vi "Is Index Visited.vi"(8 "error in (no error)":errorcluster, 10 "Index":i32, 11 "Search in":refnum<class "Search.lvclass">) -> (0 "error out":errorcluster, 2 "Visited?":bool, 3 "Search out":refnum<class "Search.lvclass">)   [LabVIEW 2016, in "Better Search.lvlib" / "Search.lvclass"]
uses:
  Search.lvclass
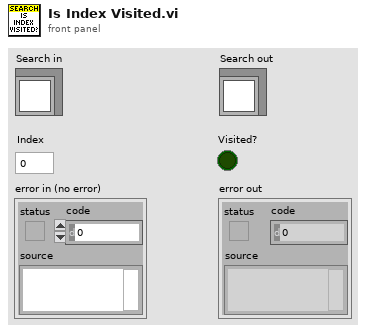
[diagram p1: front panel]
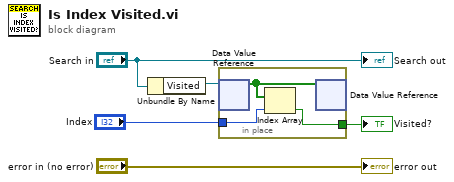
[diagram p0: block diagram]
diagram:
  n1 = Unbundle By Name("Search in") -> ("Visited"=w4:refnum<data-value>)
  n2 = in-place {
    in-place-border: "Index" -> [w7]
    in-place-border: [w6] -> w1
    n3 = in-place-dvr #1(w4) -> (w8:bool[])  [unwired: 1 out]
    n4 = Index Array(array=w8, index=w7) -> (element=w6:bool)
    n5 = in-place-dvr #1(w8) -> ()  [unwired: 2 out]
  }
  "Visited?" <- w1
  "error out" <- "error in (no error)"
  "Search out" <- "Search in"
